vi "Untitled 5 (SubVI).vi"(0 "Numeric in":i32, 5 "CamSettings":T1={"Cam 0"={"position"=0.0, "pixelsize"=0.0, "start"=0.0, "end"=0.0, "center"=0.0, "Lens"=enum."FL1-f8x08", "Forward"=enum."off", "Spec_Calib_file 2"=path "Y:/100TWdata/ESMCalib/datFwd.txt", "map"=path "Y:/100TWdata/ESMCalib/mapFwd.txt", "y size"=0, "UserROI"={"Width"={"Value"=0.0, "Min"=0.0, "Max"=0.0, "StepSize"=0.0, "Tolerance"=0.0, "ValueActual"=0.0}, "Hight"={"Value"=0.0, "Min"=0.0, "Max"=0.0, "StepSize"=0.0, "Tolerance"=0.0, "ValueActual"=0.0}, "OffsetX"={"Value"=0.0, "Min"=0.0, "Max"=0.0, "StepSize"=0.0, "Tolerance"=0.0, "ValueActual"=0.0}, "OffsetY"={"Value"=0.0, "Min"=0.0, "Max"=0.0, "StepSize"=0.0, "Tolerance"=0.0, "ValueActual"=0.0}}, "CamMaxPixel"={"X"=0, "Y"=0}, "CamROI"={"Width"=0.0, "Hight"=0.0, "OffsetX"=0.0, "OffsetY"=0.0}}, "Cam 1"={"position"=0.0, "pixelsize"=0.0, "start"=0.0, "end"=0.0, "center"=0.0, "Lens"=enum."FL1-f8x08", "Forward"=enum."off", "Spec_Calib_file 2"=path "Y:/100TWdata/ESMCalib/datFwd.txt", "map"=path "Y:/100TWdata/ESMCalib/mapFwd.txt", "y size"=0, "UserROI"={"Width"={"Value"=0.0, "Min"=0.0, "Max"=0.0, "StepSize"=0.0, "Tolerance"=0.0, "ValueActual"=0.0}, "Hight"={"Value"=0.0, "Min"=0.0, "Max"=0.0, "StepSize"=0.0, "Tolerance"=0.0, "ValueActual"=0.0}, "OffsetX"={"Value"=0.0, "Min"=0.0, "Max"=0.0, "StepSize"=0.0, "Tolerance"=0.0, "ValueActual"=0.0}, "OffsetY"={"Value"=0.0, "Min"=0.0, "Max"=0.0, "StepSize"=0.0, "Tolerance"=0.0, "ValueActual"=0.0}}, "CamMaxPixel"={"X"=0, "Y"=0}, "CamROI"={"Width"=0.0, "Hight"=0.0, "OffsetX"=0.0, "OffsetY"=0.0}}, "Cam 2"={"position"=0.0, "pixelsize"=0.0, "start"=0.0, "end"=0.0, "center"=0.0, "Lens"=enum."FL1-f8x08", "Forward"=enum."off", "Spec_Calib_file 2"=path "Y:/100TWdata/ESMCalib/datFwd.txt", "map"=path "Y:/100TWdata/ESMCalib/mapFwd.txt", "y size"=0, "UserROI"={"Width"={"Value"=0.0, "Min"=0.0, "Max"=0.0, "StepSize"=0.0, "Tolerance"=0.0, "ValueActual"=0.0}, "Hight"={"Value"=0.0, "Min"=0.0, "Max"=0.0, "StepSize"=0.0, "Tolerance"=0.0, "ValueActual"=0.0}, "OffsetX"={"Value"=0.0, "Min"=0.0, "Max"=0.0, "StepSize"=0.0, "Tolerance"=0.0, "ValueActual"=0.0}, "OffsetY"={"Value"=0.0, "Min"=0.0, "Max"=0.0, "StepSize"=0.0, "Tolerance"=0.0, "ValueActual"=0.0}}, "CamMaxPixel"={"X"=0, "Y"=0}, "CamROI"={"Width"=0.0, "Hight"=0.0, "OffsetX"=0.0, "OffsetY"=0.0}}, "Cam 3"={"position"=0.0, "pixelsize"=0.0, "start"=0.0, "end"=0.0, "center"=0.0, "Lens"=enum."FL1-f8x08", "Forward"=enum."off", "Spec_Calib_file 2"=path "Y:/100TWdata/ESMCalib/datFwd.txt", "map"=path "Y:/100TWdata/ESMCalib/mapFwd.txt", "y size"=0, "UserROI"={"Width"={"Value"=0.0, "Min"=0.0, "Max"=0.0, "StepSize"=0.0, "Tolerance"=0.0, "ValueActual"=0.0}, "Hight"={"Value"=0.0, "Min"=0.0, "Max"=0.0, "StepSize"=0.0, "Tolerance"=0.0, "ValueActual"=0.0}, "OffsetX"={"Value"=0.0, "Min"=0.0, "Max"=0.0, "StepSize"=0.0, "Tolerance"=0.0, "ValueActual"=0.0}, "OffsetY"={"Value"=0.0, "Min"=0.0, "Max"=0.0, "StepSize"=0.0, "Tolerance"=0.0, "ValueActual"=0.0}}, "CamMaxPixel"={"X"=0, "Y"=0}, "CamROI"={"Width"=0.0, "Hight"=0.0, "OffsetX"=0.0, "OffsetY"=0.0}}}, 7 "X size":dbl, 9 "emptyZArrayforreshape in":T8, 12 "Cam 1":T9) -> (1 "Array 2":dbl[](array[numeric]), 2 "Array":i32[](array[numeric]), 3 "min value":dbl, 4 "Numeric out":i32, 6 "Array 3":i32[](array[numeric]), 8 "emptyZArrayforreshape out":T8, 10 "Array 4":i32[][](array[numeric]), 13 "Array 7":i32[](array[numeric]), 14 "Array 5":i32[][](array[numeric]), 15 "Array 6":i32[](array[numeric]))   [LabVIEW 2013, in "MagAnalysis_Online.lvclass"]
uses:
  MagAnalysis_Online.lvclass
  emptyArrayCamX_TypDef.ctl
  emptyArray_TYpDEf.ctl
  OnOffTypeDef.ctl
  CamSettingSUB_TypDEf.ctl
  CamSettings_Typdef.ctl
  support0/CamAndObj_TypDEf.ctl
  source/Device Driver/shared/numericVariable_TypeDef.ctl
  source/Device Driver/BaseDriver/BaseDriver.lvclass
  userROI.ctl
  CamRoiTypDef.ctl
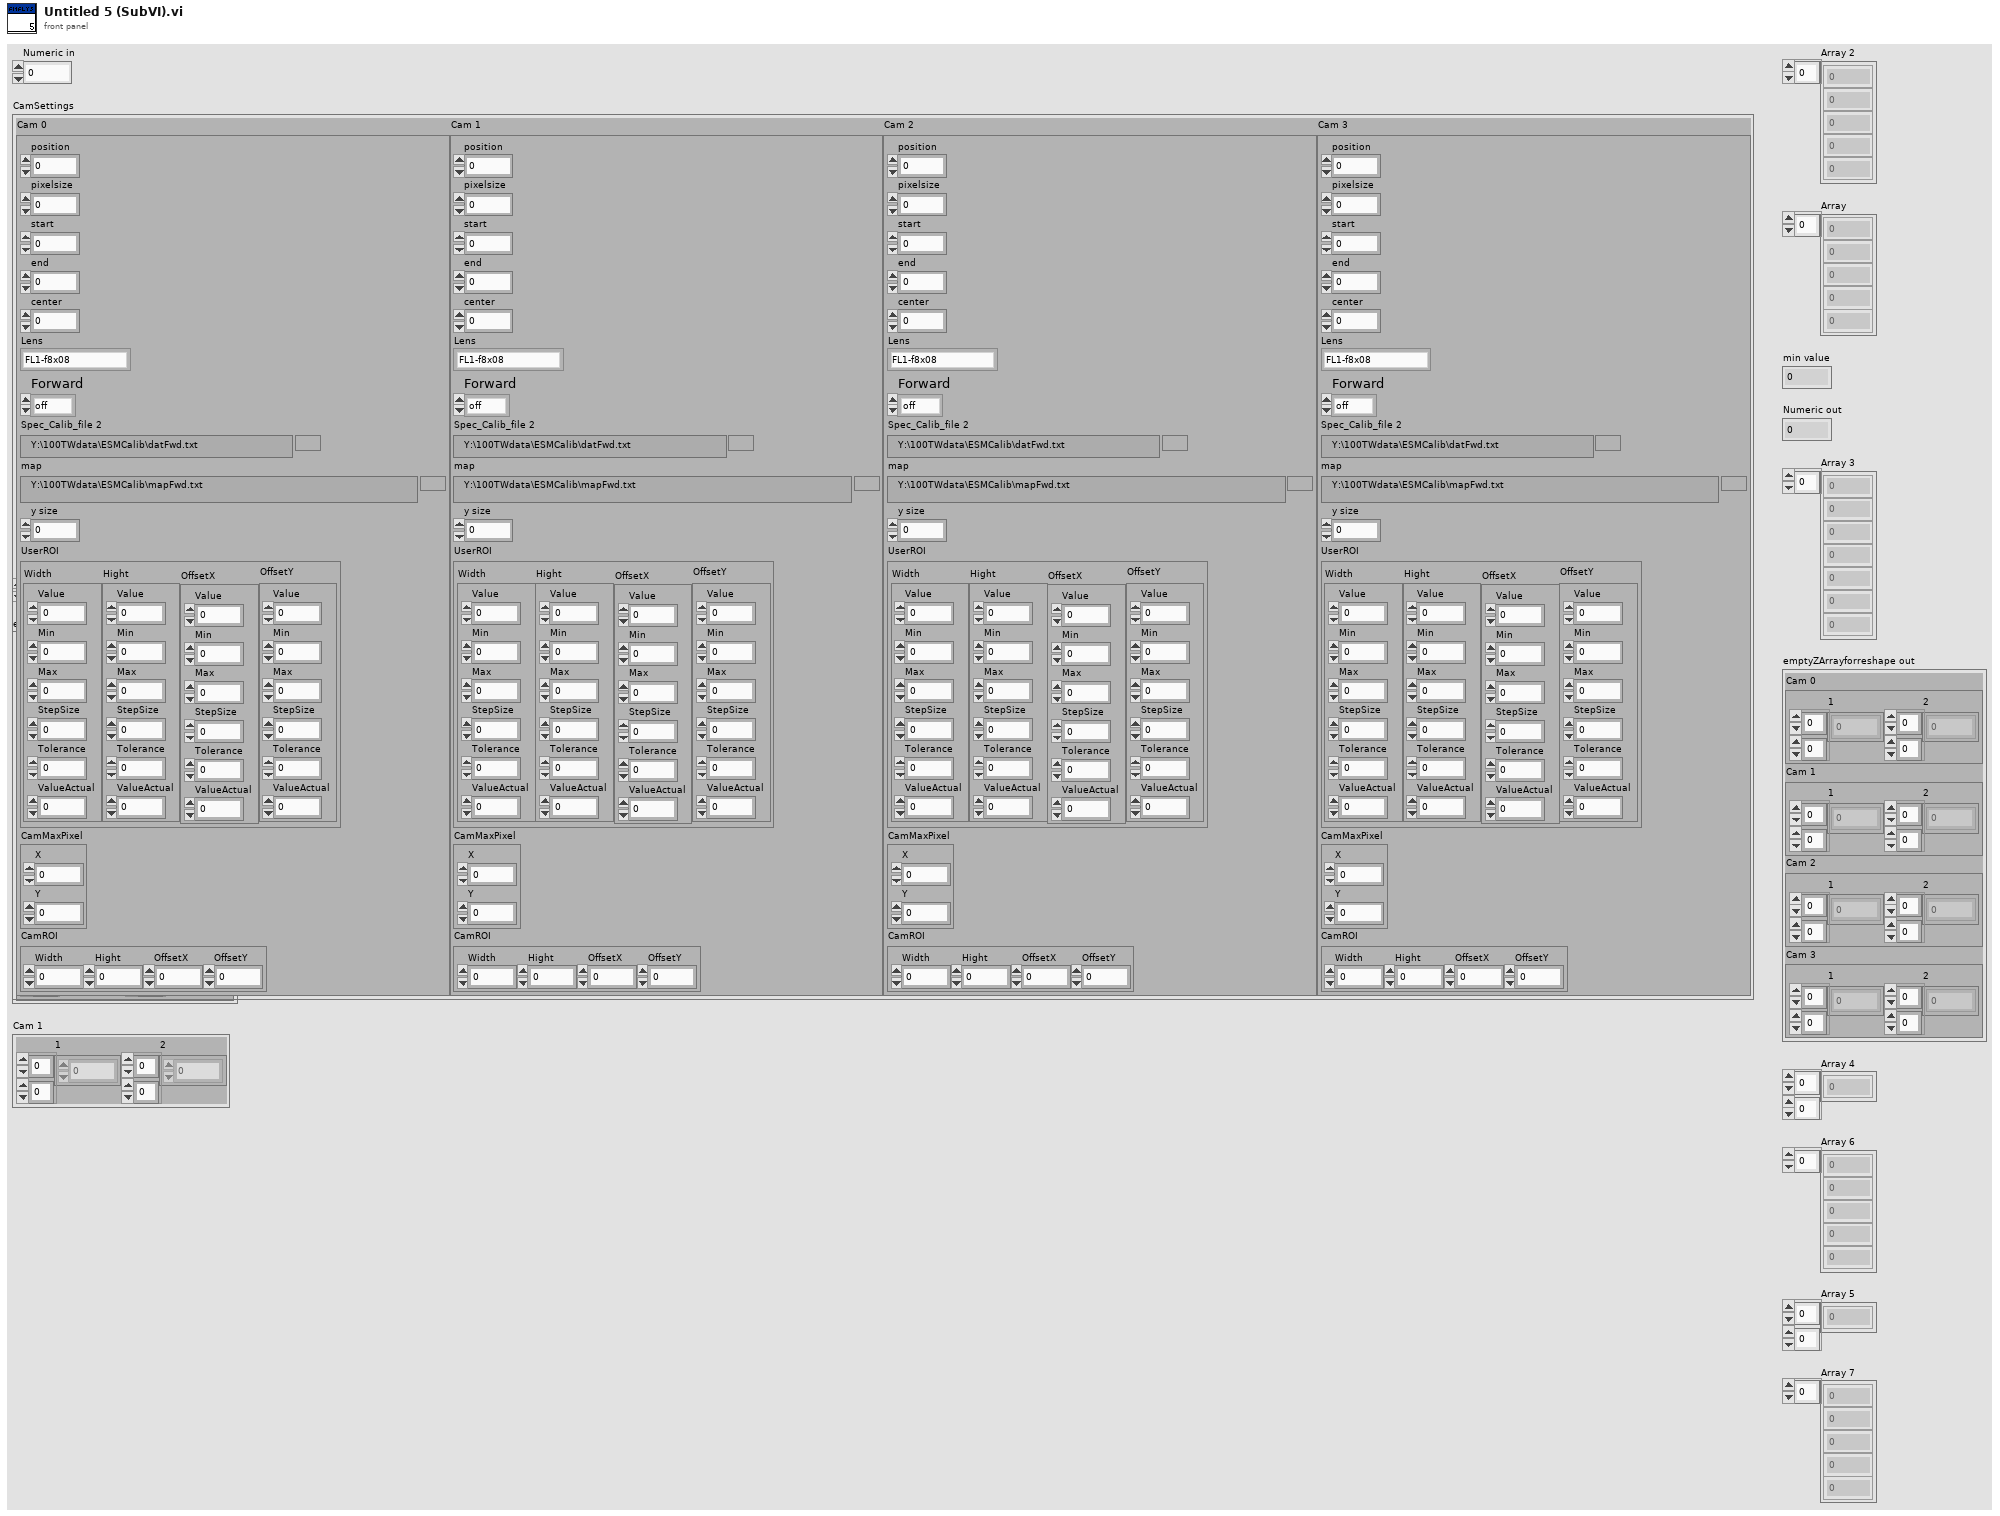
[diagram p1: front panel]
types:
  T1 = typedef "CamSettings_Typdef.ctl" = cluster{"Cam 0":T2, "Cam 1":T2, "Cam 2":T2, "Cam 3":T2}
  T2 = typedef "CamSettingSUB_TypDEf.ctl" = cluster{"position":dbl, "pixelsize":dbl, "start":dbl, "end":dbl, "center":dbl, "Lens":T3, "Forward":T4, "Spec_Calib_file 2":path, "map":path, "y size":i32, "UserROI":T5, "CamMaxPixel":cluster{"X":i32, "Y":i32}, "CamROI":T7}
  T3 = typedef "CamAndObj_TypDEf.ctl" = enum16{"FL1-f8x08", "FL1-f8x06", "FL1-f8", "ch300-f50", "FL2G-f8", "FL3M14-f8", "FL3M14-f8x08", "FL3M14-f8x08(2x2)"}
  T4 = typedef "OnOffTypeDef.ctl" = enum16{"off", "on"}
  T5 = typedef "userROI.ctl" = cluster{"Width":T6, "Hight":T6, "OffsetX":T6, "OffsetY":T6}
  T6 = typedef "BaseDriver.lvclass/numericVariable_TypeDef.ctl" = cluster{"Value":dbl, "Min":dbl, "Max":dbl, "StepSize":dbl, "Tolerance":dbl, "ValueActual":dbl}
  T7 = typedef "CamRoiTypDef.ctl" = cluster{"Width":dbl, "Hight":dbl, "OffsetX":dbl, "OffsetY":dbl}
  T8 = typedef "emptyArray_TYpDEf.ctl" = cluster{"Cam 0":T9, "Cam 1":T9, "Cam 2":T9, "Cam 3":T9}
  T9 = typedef "emptyArrayCamX_TypDef.ctl" = cluster{"1":dbl[][], "2":dbl[][]}
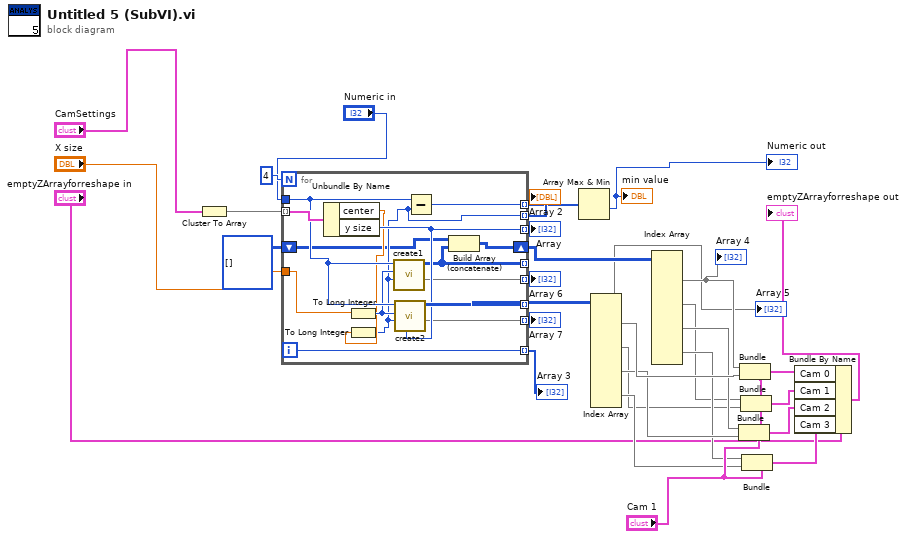
[diagram p0: block diagram]
diagram:
  n1 = Cluster To Array(cluster="CamSettings") -> (array=w2:T2[])
  n2 = for {
    N: 4 -> [_]
    tunnel: w2 -> [w45] mode=indexing
    tunnel: "Numeric in" -> [w43]
    tunnel: [w44] -> w1 mode=indexing
    tunnel: "X size" -> [w37]
    tunnel: [w33] -> _ mode=indexing
    tunnel: [w42] -> w7 mode=indexing
    tunnel: [w41] -> w14 mode=indexing
    tunnel: [w34] -> w19 mode=indexing
    tunnel: [w40] -> w22 mode=indexing
    tunnel: [w39] -> w26 mode=indexing
    tunnel: [w38] -> w27 mode=indexing
    shift-right: [w32] -> w30
    shift-left: i32[][][] [] -> [w31]
    i -> [w40]
    n3 = Unbundle By Name(w45) -> ("center"=w35:dbl, "y size"=w41:i32)
    n4 = To Long Integer(number=w37) -> (32bit integer=w36:i32)
    n5 = To Long Integer(number=w35) -> (32bit integer=w34:i32)
    n6 = call "create1.vi"("center"=w34, "X size"=w36, "max Y size"=w43) -> (1:w39, "Array"=w33:i32[][])  [unwired: 6 in, 1 out]
    n7 = call "create2.vi"("actual y size"=w41, "center"=w34, "X size"=w36, "max Y size"=w43) -> (1:w38, "Array"=w42:i32[][])  [unwired: 5 in, 1 out]
    n8 = Subtract(x=w43, y=w34) -> (x-y=w44:i32)
    n9 = Build Array (concatenate)(w31, w33) -> (w32:i32[][][])
  }
  "Array" <- w14
  "Array 2" <- w19
  "Array 3" <- w22
  "Array 6" <- w26
  "Array 7" <- w27
  n10 = Array Max & Min(array=w1) -> (min value=→"min value" →"Numeric out":i32)  [unwired: 3 out]
  n11 = Index Array(array=w7) -> (element #1=w24:i32[][], element #2=w16:i32[][], element #3=w20:i32[][], element #4=w18:i32[][])  [unwired: 12 in]
  "Array 5" <- w24
  n12 = Index Array(array=w30) -> (element #1=w28:i32[][], element #2=w15:i32[][], element #3=w21:i32[][], element #4=w17:i32[][])  [unwired: 12 in]
  "Array 4" <- w28
  n13 = Bundle(cluster="Cam 1", "1"=w21, "2"=w20) -> (w11:T9)
  n14 = Bundle(cluster="Cam 1", "1"=w28, "2"=w24) -> (w9:T9)
  n15 = Bundle(cluster="Cam 1", "1"=w15, "2"=w16) -> (w10:T9)
  n16 = Bundle(cluster="Cam 1", "1"=w17, "2"=w18) -> (w12:T9)
  n17 = Bundle By Name(cluster="emptyZArrayforreshape in", "Cam 0"=w9, "Cam 1"=w10, "Cam 2"=w11, "Cam 3"=w12) -> (→"emptyZArrayforreshape out":T8)
